vi "_Get Monitor Center Point.vi"() -> (3 "Center":cluster{"x":i32, "y":i32})   [LabVIEW 2017]
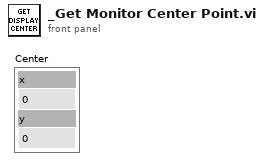
[diagram p1: front panel]
types:
  T1 = typedef "LVRectTypeDef.ctl" = cluster{"Left":i16, "Top":i16, "Right":i16, "Bottom":i16}
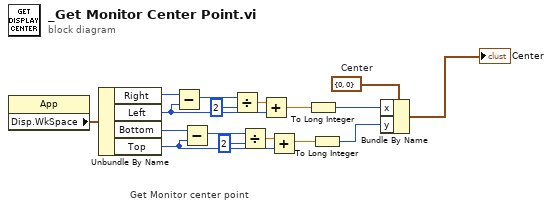
[diagram p0: block diagram]
diagram:
  w7 = cluster{"x":i32, "y":i32} {"x"=0, "y"=0}  # Center
  # "Get Monitor center point"
  n1 = property class="App"() -> ("Disp.WkSpace"=w1:T1)  [unwired: 2 in, 2 out]
  n2 = Unbundle By Name(w1) -> ("Right"=w15:i16, "Left"=w13:i16, "Bottom"=w9:i16, "Top"=w8:i16)
  n3 = Subtract(x=w15, y=w13) -> (x-y=w14:i16)
  n4 = Subtract(x=w9, y=w8) -> (x-y=w12:i16)
  n5 = Divide(x=w14, y=i16 2) -> (x/y=w16:dbl)
  n6 = Divide(x=w12, y=i16 2) -> (x/y=w11:dbl)
  n7 = Add(x=w16, y=w13) -> (x+y=w6:dbl)
  n8 = Add(x=w11, y=w8) -> (x+y=w5:dbl)
  n9 = To Long Integer(number=w6) -> (32bit integer=w4:i32)
  n10 = To Long Integer(number=w5) -> (32bit integer=w3:i32)
  n11 = Bundle By Name(cluster=w7, "x"=w4, "y"=w3) -> (→"Center":cluster{"x":i32, "y":i32})
